vi "DamnYankeeHindbrainRemoteControlSense.vi"(10 "Notifier References":T9, 11 "IO Cluster":T1) -> (0 "Error out":errorcluster)   [LabVIEW 2013]
doc: "This VI reads the remote control data that is coming in and continually updates what the boat thinks the controller is doing. It's in a separate while loop from the rest of the Sense data because the direct reading of PWM signals requires a somewhat consistent time-step.\n\nEric Schneider, May 2014"
uses:
  Data/TypeDefs/Notifiers.ctl
  Data/TypeDefs/UTM Location.ctl
  Data/TypeDefs/Sail Set Suggestions.ctl
  Data/TypeDefs/Rudder Set Suggestions.ctl
  Data/TypeDefs/OverrideInformation.ctl
  Data/TypeDefs/OverrideMode.ctl
  Data/TypeDefs/MotorSetup.ctl
  Data/TypeDefs/DynamixelSetupInfo.ctl
  Data/TypeDefs/AirmarStatus.ctl
  Data/TypeDefs/HardwareOnline.ctl
  Data/TypeDefs/DynamixelCycleTracker.ctl
  Data/TypeDefs/RC Input Values.ctl
  Data/TypeDefs/DamnYankeeIOPorts.ctl
  <vilib>/myRIO/Instrument Drivers/Onboard IO/DIO/typedefs/DIO Reference.ctl
  <vilib>/myRIO/Common/Instrument Driver Framework/Utilities/typedefs/myRIO Generic Hardware Reference.ctl
  <vilib>/myRIO/Common/Instrument Driver Framework/Utilities/typedefs/Hardware Version Enum.ctl
  <vilib>/myRIO/Common/Instrument Driver Framework/Utilities/typedefs/myRIO v1.0 Reference.ctl
  <vilib>/myRIO/Common/Instrument Driver Framework/Utilities/typedefs/Generic FPGA Reference.ctl
  <vilib>/myRIO/Common/Instrument Driver Framework/myRIO v1.0/DIO/typedefs/DIO Channels List.ctl
  <vilib>/myRIO/Common/Instrument Driver Framework/myRIO v1.0/DIO/typedefs/DIO Channels Enum.ctl
  <vilib>/Utility/error.llb/Error Cluster From Error Code.vi
  <vilib>/myRIO/Common/Instrument Driver Framework/myRIO v1.0/DIO/vis/myRIO v1.0 Read DIO.vi
  <vilib>/myRIO/Instrument Drivers/Onboard IO/DIO/DIO.lvlib
panel:
  out "Rudder Chart":dbl(graph)
  out "Sail Chart":dbl(graph)
  out "Switch Chart":dbl(graph)
  out "Switch Signal Chart":i16(graph)
  out "Switch value":dbl
  out "Sail value":dbl
  out "Rudder value":dbl
  # "Debugging information"
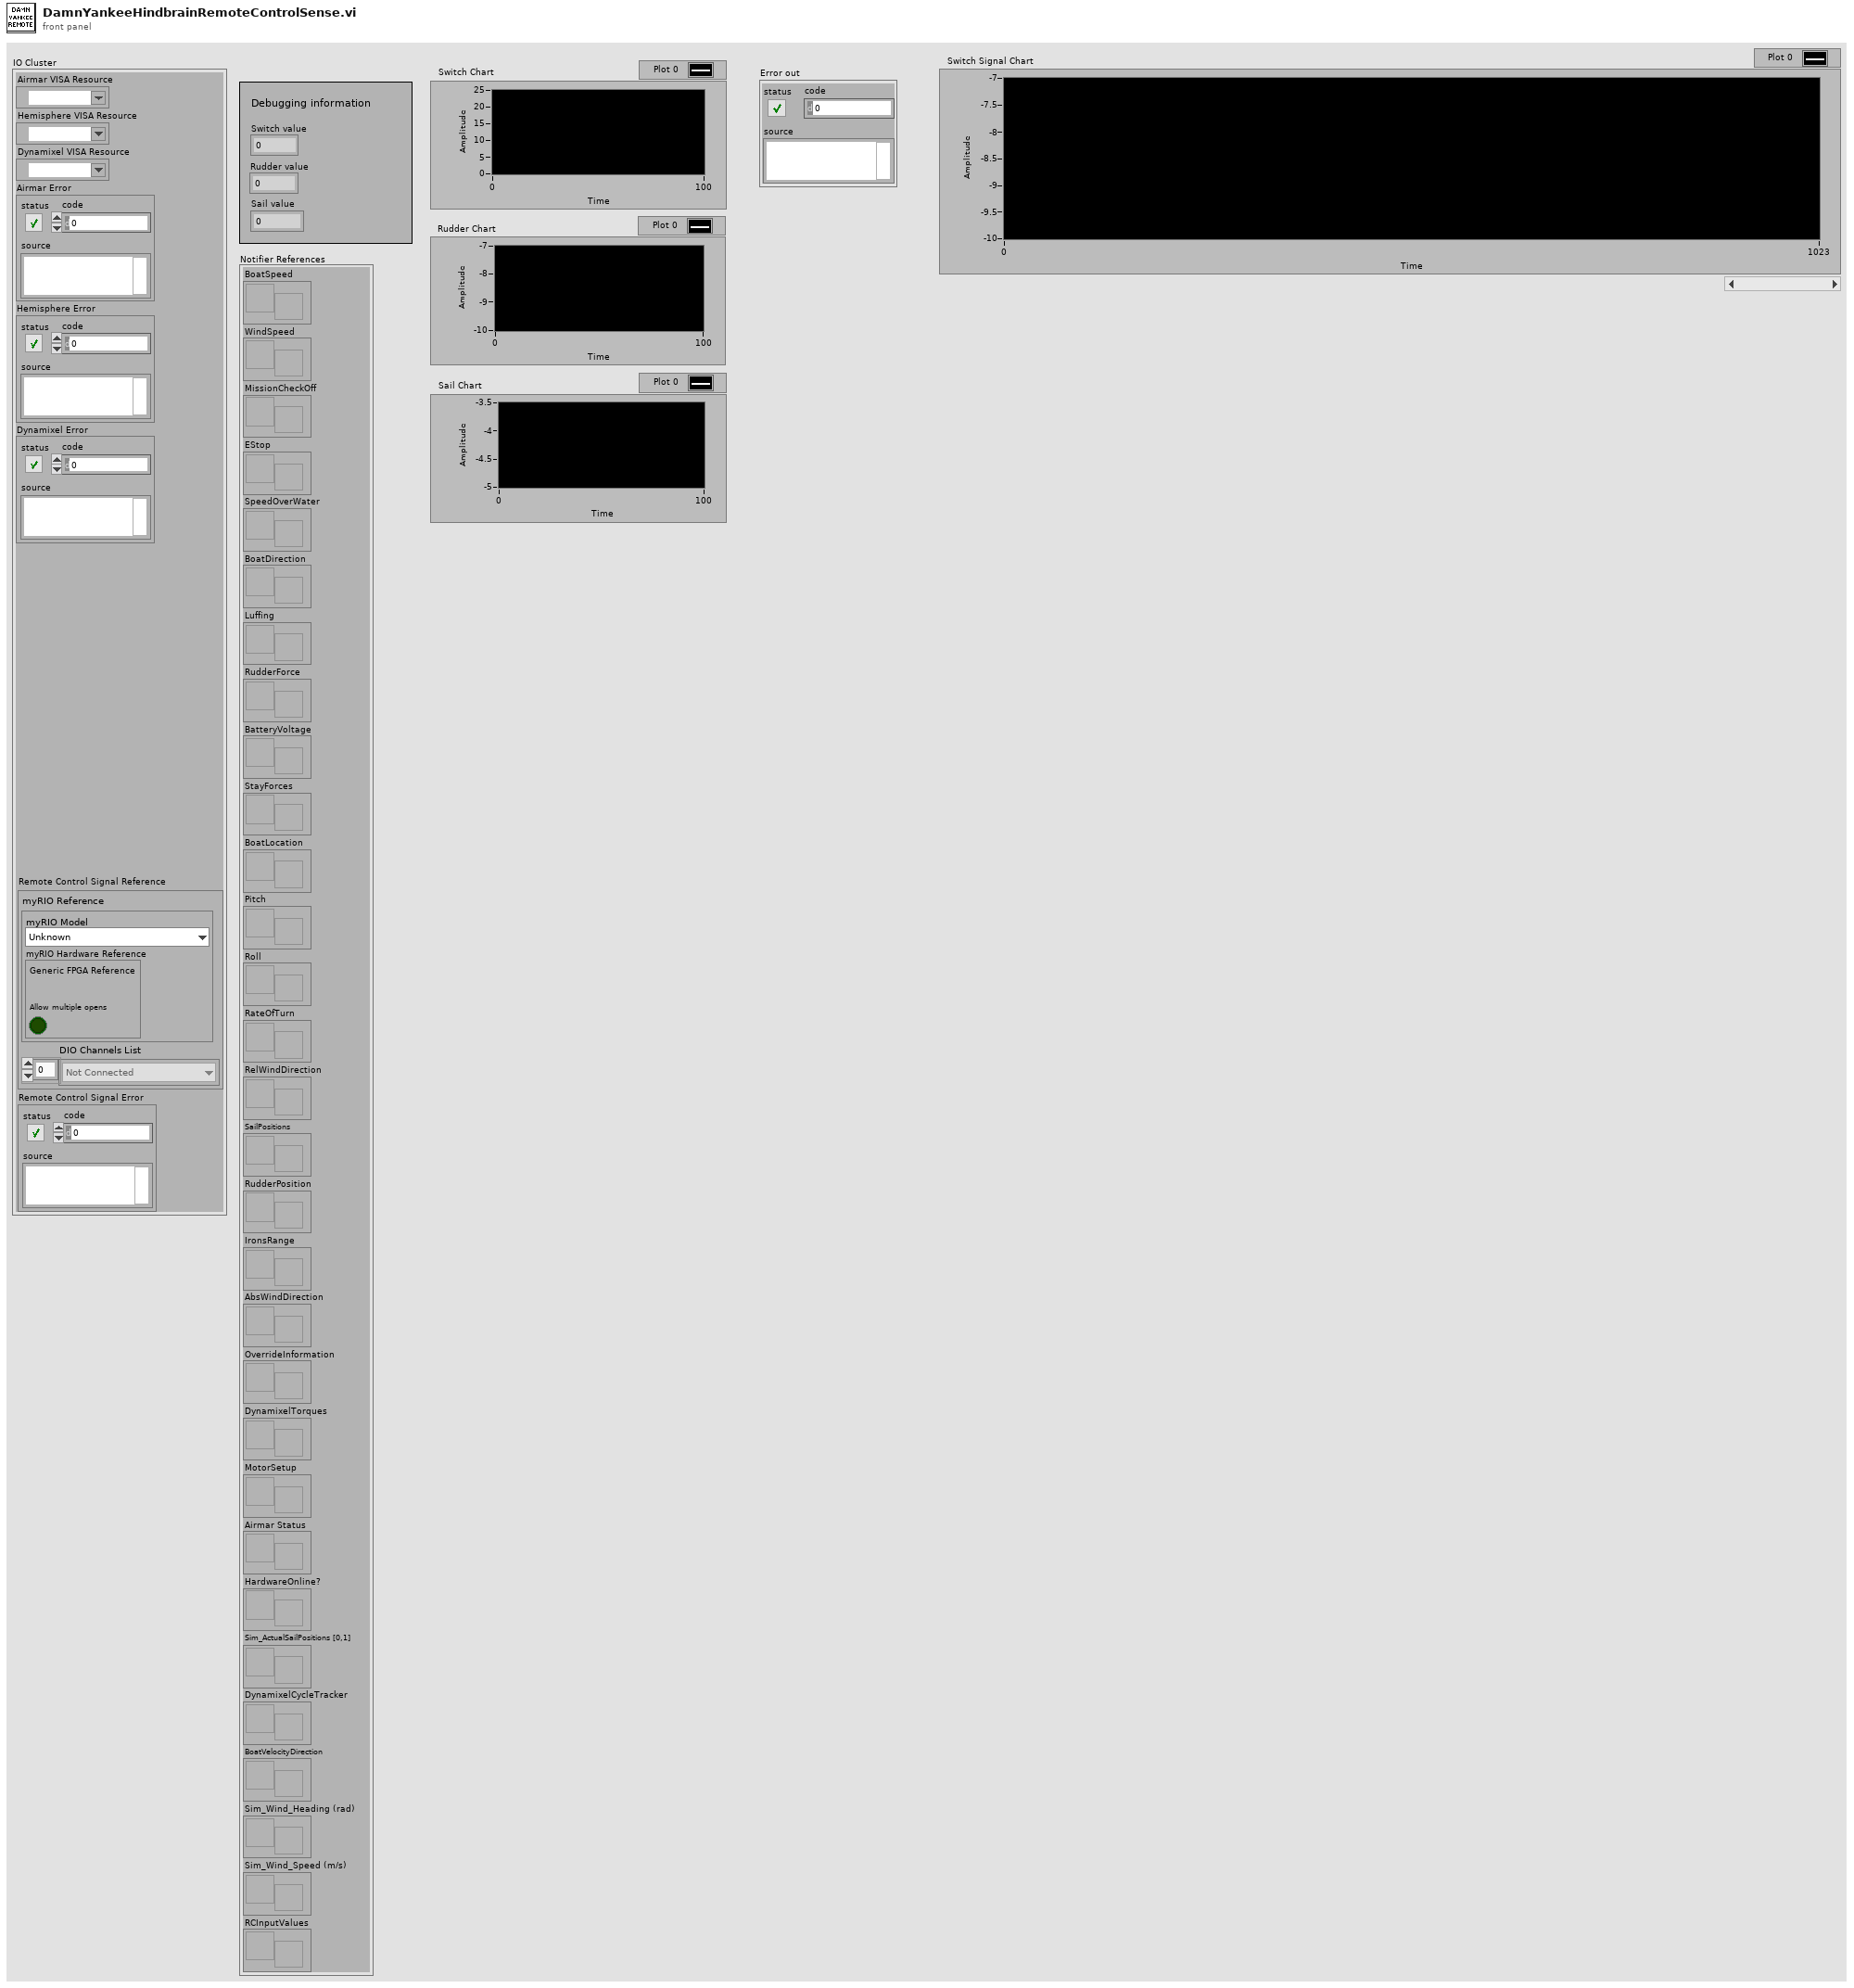
[diagram p1: front panel]
types:
  T1 = typedef "DamnYankeeIOPorts.ctl" = cluster{"Airmar VISA Resource":refnum<visa-resource-name>, "Hemisphere VISA Resource":refnum<visa-resource-name>, "Dynamixel VISA Resource":refnum<visa-resource-name>, "Airmar Error":errorcluster, "Hemisphere Error":errorcluster, "Dynamixel Error":errorcluster, "Remote Control Signal Reference":T2, "Remote Control Signal Error":errorcluster}
  T2 = typedef "DIO.lvlib/DIO Reference.ctl" = cluster{"myRIO Reference":T3, "DIO Channels List":T7}
  T3 = typedef "myRIO Generic Hardware Reference.ctl" = cluster{"myRIO Model":T4, "myRIO Hardware Reference":T5}
  T4 = typedef "Hardware Version Enum.ctl" = enum16{"Unknown", "myRIO-1900", "myRIO-1950"}
  T5 = typedef "myRIO v1.0 Reference.ctl" = cluster{"Generic FPGA Reference":T6, "Allow multiple opens":bool}
  T6 = typedef "Generic FPGA Reference.ctl" = refnum<k20>
  T7 = typedef "DIO Channels List.ctl" = T8[]
  T8 = typedef "DIO Channels Enum.ctl" = enum16{"Not Connected", "C/DIO0", "C/DIO1", "C/DIO2", "C/DIO3", "C/DIO4", "C/DIO5", "C/DIO6", "C/DIO7", "A/DIO0", "A/DIO1", "A/DIO2", "A/DIO3", "A/DIO4", "A/DIO5", "A/DIO6", "A/DIO7", "A/DIO8", "A/DIO9", "A/DIO10", "A/DIO11", "A/DIO12", "A/DIO13", "A/DIO14", "A/DIO15", "B/DIO0", "B/DIO1", "B/DIO2", "B/DIO3", "B/DIO4", "B/DIO5", "B/DIO6", "B/DIO7", "B/DIO8", "B/DIO9", "B/DIO10", "B/DIO11", "B/DIO12", "B/DIO13", "B/DIO14", "B/DIO15", "LED0", "LED1", "LED2", "LED3", "Button0"}
  T9 = typedef "Notifiers.ctl" = cluster{"BoatSpeed":refnum<notifier>, "WindSpeed":refnum<notifier>, "MissionCheckOff":refnum<notifier>, "EStop":refnum<notifier>, "SpeedOverWater":refnum<notifier>, "BoatDirection":refnum<notifier>, "Luffing":refnum<notifier>, "RudderForce":refnum<notifier>, "BatteryVoltage":refnum<notifier>, "StayForces":refnum<notifier>, "BoatLocation":refnum<notifier>, "Pitch":refnum<notifier>, "Roll":refnum<notifier>, "RateOfTurn":refnum<notifier>, "RelWindDirection":refnum<notifier>, "SailPositions":refnum<notifier>, "RudderPosition":refnum<notifier>, "IronsRange":refnum<notifier>, "AbsWindDirection":refnum<notifier>, "OverrideInformation":refnum<notifier>, "DynamixelTorques":refnum<notifier>, "MotorSetup":refnum<notifier>, "Airmar Status":refnum<notifier>, "HardwareOnline?":refnum<notifier>, "Sim_ActualSailPositions [0,1]":refnum<notifier>, "DynamixelCycleTracker":refnum<notifier>, "BoatVelocityDirection":refnum<notifier>, "Sim_Wind_Heading (rad)":refnum<notifier>, "Sim_Wind_Speed (m/s)":refnum<notifier>, "RCInputValues":refnum<notifier>}
  T10 = typedef "RC Input Values.ctl" = cluster{"RC Switch Value":dbl, "Sail setpoints":T11, "Rudder Setpoint":T12}
  T11 = typedef "Sail Set Suggestions.ctl" = cluster{"MainSailSuggestion":dbl, "JibSailSuggestion":dbl}
  T12 = typedef "Rudder Set Suggestions.ctl" = dbl
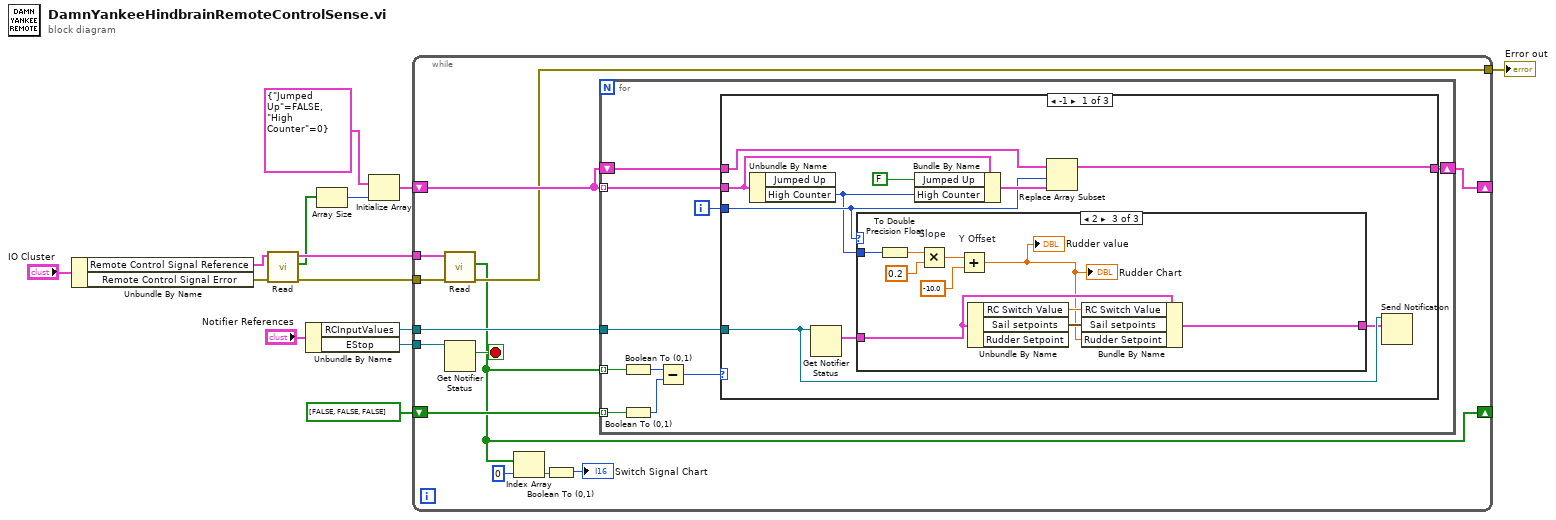
[diagram p0: block diagram]
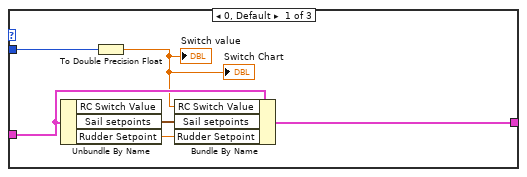
[diagram p2: hidden frame]
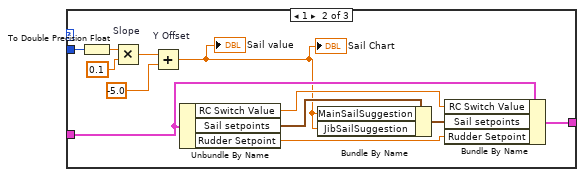
[diagram p3: hidden frame]
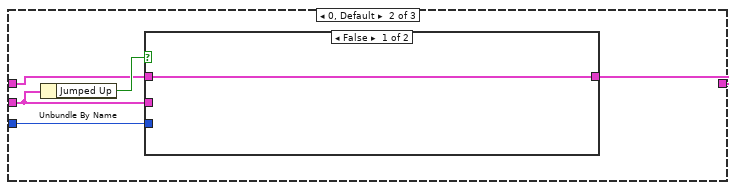
[diagram p4: hidden frame]
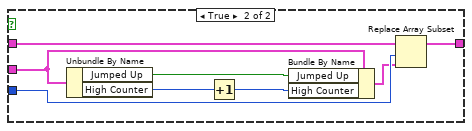
[diagram p5: hidden frame]
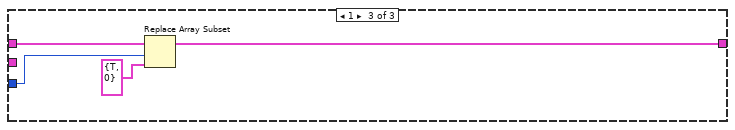
[diagram p6: hidden frame]
diagram:
  n1 = Unbundle By Name("IO Cluster") -> ("Remote Control Signal Reference"=w7:T2, "Remote Control Signal Error"=w6:errorcluster)
  n2 = call <vilib>:"Read.vi"("error in (no error)"=w6, "DIO Ref In"=w7) -> ("error out"=w4:errorcluster, "Values"=w3:bool[], "DIO Ref Out"=w5:T2)  [unwired: 7 in]
  n3 = Unbundle By Name("Notifier References") -> ("RCInputValues"=w12:refnum<notifier>, "EStop"=w11:refnum<notifier>)
  n4 = Array Size(array=w3) -> (size(s)=w2:i32)
  n5 = Initialize Array(cluster{"Jumped Up":bool, "High Counter":i32} {"Jumped Up"=FALSE, "High Counter"=0}, w2) -> (w9:cluster{"Jumped Up":bool, "High Counter":i32}[])
  n6 = while {
    tunnel: w11 -> [w27]
    tunnel: w12 -> [w20]
    tunnel: w5 -> [w25]
    tunnel: w4 -> [w24]
    shift-right: [w18] -> _
    shift-left: bool[] [FALSE, FALSE, FALSE] ("Values") -> [w23]
    shift-right: [w21] -> _
    shift-left: w9 -> [w22]
    tunnel: [w19] -> w1
    stop <- w26 stop-if-true
    n7 = call <vilib>:"Read.vi"("error in (no error)"=w24, "DIO Ref In"=w25) -> ("error out"=w19:errorcluster, "Values"=w18:bool[])  [unwired: 7 in, 1 out]
    n8 = Get Notifier Status(notifier=w27) -> (current notification=w26:bool)  [unwired: 1 in, 4 out]
    n9 = Index Array(array=w18, index=0) -> (element=w16:bool)
    n10 = Boolean To (0,1)(Boolean=w16) -> (0, 1=→"Switch Signal Chart":i16)
    n11 = for {
      tunnel: w18 -> [w36] mode=indexing
      tunnel: w23 -> [w37] mode=indexing
      tunnel: w22 -> [w32] mode=indexing
      shift-right: [w29] -> w21
      shift-left: w22 -> [w31]
      tunnel: w20 -> [w28]
      i -> [w30]
      n12 = Boolean To (0,1)(Boolean=w36) -> (0, 1=w34:i16)
      n13 = Boolean To (0,1)(Boolean=w37) -> (0, 1=w33:i16)
      n14 = Subtract(x=w34, y=w33) -> (x-y=w35:i16)
      n15 = case shown="-1" w35 {
        tunnel: w32 -> [w45 w79 _]
        tunnel: w31 -> [w46 w78 w93]
        tunnel: w30 -> [w42 w77 w92]
        tunnel: [w43 w76 w91] -> w29
        tunnel: w28 -> [w40 _ _]
        frame -1 {
          n16 = Unbundle By Name(w45) -> ("High Counter"=w38:i32)  [unwired: 1 out]
          n17 = Get Notifier Status(notifier=w40) -> (current notification=w41:T10)  [unwired: 1 in, 4 out]
          n18 = case shown="2" w42 {
            tunnel: w41 -> [w51 w63 w73]
            tunnel: [w50 w62 w72] -> w39
            tunnel: w38 -> [w49 w55 w71]
            frame 0, Default {
              n19 = Unbundle By Name(w51) -> ("Sail setpoints"=w53:T11, "Rudder Setpoint"=w52:T12)  [unwired: 1 out]
              n20 = To Double Precision Float(number=w49) -> (double precision float=w48:dbl)
              "Switch value" <- w48
              "Switch Chart" <- w48
              n21 = Bundle By Name(cluster=w51, "RC Switch Value"=w48, "Sail setpoints"=w53, "Rudder Setpoint"=w52) -> (w50:T10)
            }
            frame 1 {
              n22 = To Double Precision Float(number=w55) -> (double precision float=w59:dbl)
              n23 = Multiply "Slope"(x=w59, y=0.1) -> (x*y=w57:dbl)
              n24 = Add "Y Offset"(x=w57, y=-5.0) -> (x+y=w54:dbl)
              "Sail value" <- w54
              "Sail Chart" <- w54
              n25 = Unbundle By Name(w63) -> ("RC Switch Value"=w65:dbl, "Sail setpoints"=w61:T11, "Rudder Setpoint"=w64:T12)
              n26 = Bundle By Name(cluster=w61, "MainSailSuggestion"=w54, "JibSailSuggestion"=w54) -> (w60:T11)
              n27 = Bundle By Name(cluster=w63, "RC Switch Value"=w65, "Sail setpoints"=w60, "Rudder Setpoint"=w64) -> (w62:T10)
            }
            frame 2 {
              n28 = To Double Precision Float(number=w71) -> (double precision float=w70:dbl)
              n29 = Multiply "Slope"(x=w70, y=0.2) -> (x*y=w68:dbl)
              n30 = Add "Y Offset"(x=w68, y=-10.0) -> (x+y=w66:dbl)
              "Rudder value" <- w66
              "Rudder Chart" <- w66
              n31 = Unbundle By Name(w73) -> ("RC Switch Value"=w74:dbl, "Sail setpoints"=w75:T11)  [unwired: 1 out]
              n32 = Bundle By Name(cluster=w73, "RC Switch Value"=w74, "Sail setpoints"=w75, "Rudder Setpoint"=w66) -> (w72:T10)
            }
          }
          n33 = Bundle By Name(cluster=w45, "Jumped Up"=FALSE, "High Counter"=w38) -> (w47:cluster{"Jumped Up":bool, "High Counter":i32})
          n34 = Replace Array Subset(array=w46, new element=w47, index=w42) -> (w43:cluster{"Jumped Up":bool, "High Counter":i32}[])
          n35 = Send Notification(notification=w39, notifier=w40) -> ()  [unwired: 1 in, 2 out]
        }
        frame 0, Default {
          n36 = Unbundle By Name(w79) -> ("Jumped Up"=w80:bool)
          n37 = case shown="False" w80 {
            tunnel: w79 -> [_ w89]
            tunnel: w78 -> [w81 w85]
            tunnel: w77 -> [_ w84]
            tunnel: [w81 w82] -> w76
            frame False {
            }
            frame True {
              n38 = Unbundle By Name(w89) -> ("Jumped Up"=w88:bool, "High Counter"=w87:i32)
              n39 = Increment(x=w87) -> (x+1=w86:i32)
              n40 = Bundle By Name(cluster=w89, "Jumped Up"=w88, "High Counter"=w86) -> (w83:cluster{"Jumped Up":bool, "High Counter":i32})
              n41 = Replace Array Subset(array=w85, new element=w83, index=w84) -> (w82:cluster{"Jumped Up":bool, "High Counter":i32}[])
            }
          }
        }
        frame 1 {
          n42 = Replace Array Subset(array=w93, new element=cluster{"Jumped Up":bool, "High Counter":i32} {"Jumped Up"=TRUE, "High Counter"=0} ("new element/subarray"), index=w92) -> (w91:cluster{"Jumped Up":bool, "High Counter":i32}[])
        }
      }
    }
  }
  "Error out" <- w1
